vi "Parse String.vi"(8 "error in (no error)":errorcluster, 10 "start at":i32, 11 "TOML String":string) -> (0 "error out":errorcluster, 2 "offset past match":i32, 3 "String":string)   [LabVIEW 2015, in "JSON.lvlib"]
uses:
  JSON.lvlib
  <vilib>/regexp/Match Regular Expression.xnode
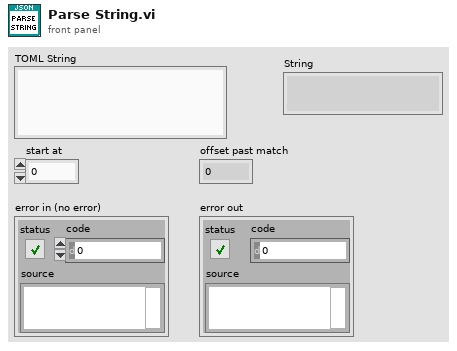
[diagram p1: front panel]
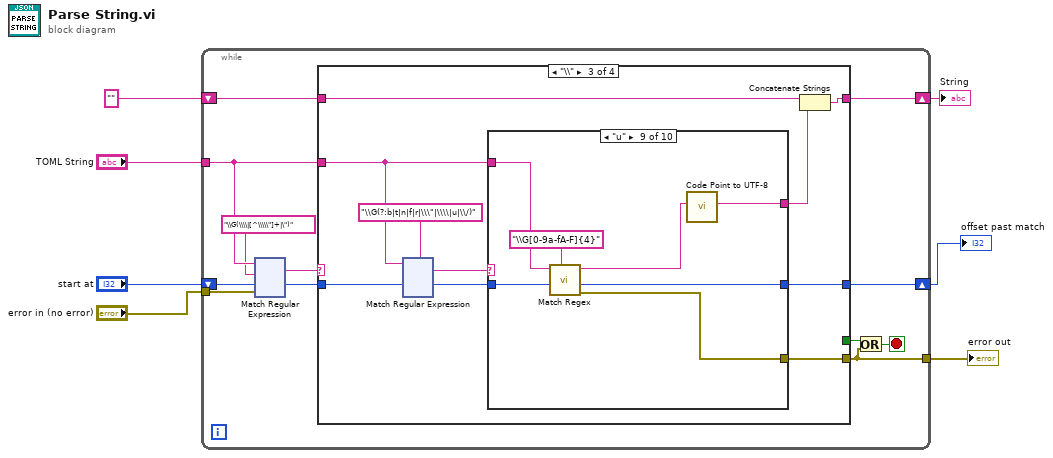
[diagram p0: block diagram]
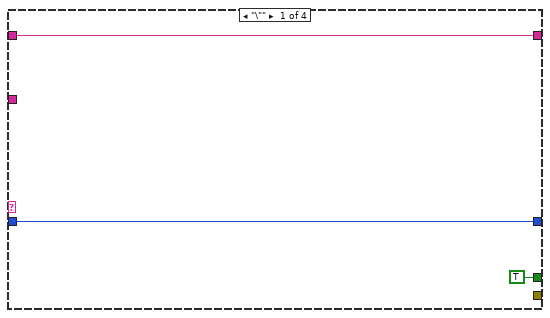
[diagram p2: hidden frame]
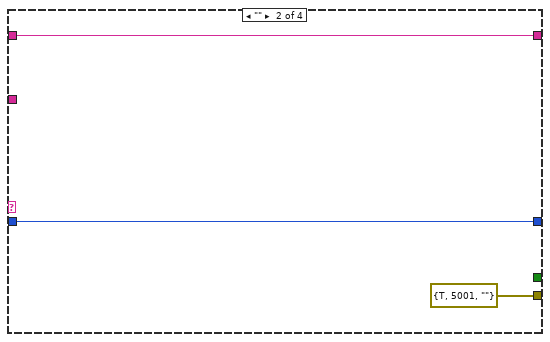
[diagram p3: hidden frame]
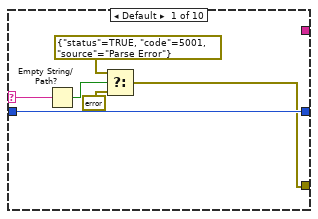
[diagram p4: hidden frame]
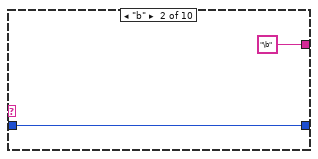
[diagram p5: hidden frame]
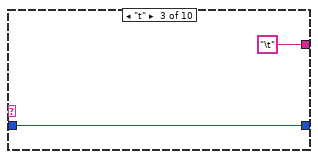
[diagram p6: hidden frame]
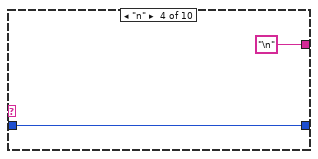
[diagram p7: hidden frame]
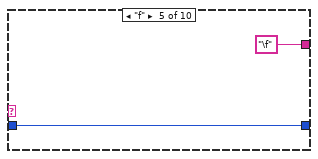
[diagram p8: hidden frame]
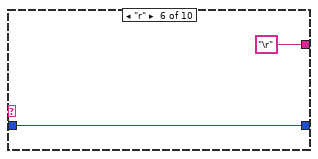
[diagram p9: hidden frame]
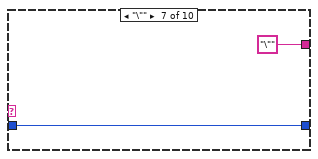
[diagram p10: hidden frame]
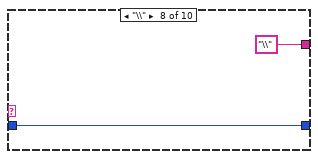
[diagram p11: hidden frame]
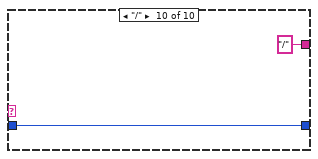
[diagram p12: hidden frame]
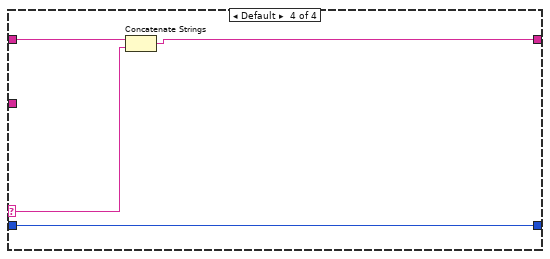
[diagram p13: hidden frame]
diagram:
  n1 = while {
    tunnel: "error in (no error)" -> [w19]
    tunnel: "TOML String" -> [w12]
    shift-right: [w17] -> w3
    shift-left: "start at" -> [w18]
    shift-right: [w15] -> w4
    shift-left: "" -> [w14]
    tunnel: [w10] -> w5
    stop <- w11 stop-if-true
    n2 = xnode "Match Regular Expression"("input string"=w12, "regular expression"="\\G(\\\\|[^\\\\\"]+|\")", "offset (0)"=w18, "error in"=w19) -> ("whole match"=w9:string, "offset past match"=w16:i32)  [unwired: 2 in, 3 out]
    n3 = case shown="\"\\\\\"" w9 {
      selector: w9 -> [_ _ _ w181]
      tunnel: [w21 w24 w31 w182] -> w17
      tunnel: w16 -> [w21 w24 w34 w182]
      tunnel: [w22 w25 w29 w179] -> w15
      tunnel: w14 -> [w22 w25 w35 w180]
      tunnel: [TRUE _ _ _] -> w13
      tunnel: w12 -> [_ _ w27 _]
      tunnel: [_ errorcluster {"status"=TRUE, "code"=5001, "source"=""} ("error constant") w32 _] -> w10
      frame "\"" {
      }
      frame "" {
      }
      frame "\\" {
        n4 = xnode "Match Regular Expression"("input string"=w27, "regular expression"="\\G(?:b|t|n|f|r|\\\"|\\\\|u|\\/)", "offset (0)"=w34) -> ("whole match"=w26:string, "offset past match"=w30:i32)  [unwired: 3 in, 3 out]
        n5 = case shown="\"u\"" w26 {
          selector: w26 -> [w40 _ _ _ _ _ _ _ _ _]
          tunnel: [w36 _ _ _ _ _ _ _ w59 _] -> w32
          tunnel: [w41 w42 w44 w46 w48 w50 w52 w54 w60 w63] -> w31
          tunnel: w30 -> [w41 w42 w44 w46 w48 w50 w52 w54 w61 w63]
          tunnel: [_ "\b" ("regular expression") "\t" ("regular expression") "\n" ("regular expression") "\f" ("regular expression") "\r" ("regular expression") "\"" ("regular expression") "\\" ("regular expression") w57 "/" ("UTF-8")] -> w28
          tunnel: w27 -> [_ _ _ _ _ _ _ _ w62 _]
          frame Default {
            n6 = Empty String/Path?(string/path=w40) -> (empty?=w39:bool)
            n7 = Select(t=errorcluster {"status"=TRUE, "code"=5001, "source"="Parse Error"} ("error constant"), s=w39, f=errorcluster {"status"=FALSE, "code"=0, "source"=""}) -> (s? t:f=w36:errorcluster)
          }
          frame "b" {
          }
          frame "t" {
          }
          frame "n" {
          }
          frame "f" {
          }
          frame "r" {
          }
          frame "\"" {
          }
          frame "\\" {
          }
          frame "u" {
            n8 = call "Match Regex.vi"("regular expression"="\\G[0-9a-fA-F]{4}", "offset"=w61, "String"=w62) -> ("error out"=w59:errorcluster, "offset past match"=w60:i32, "whole match"=w56:string)  [unwired: 5 in, 1 out]
            n9 = call "Code Point to UTF-8.vi"("Code Point"=w56) -> ("UTF-8"=w57:string)  [unwired: 10 in]
          }
          frame "/" {
          }
        }
        n10 = Concatenate Strings(w35, w28) -> (w29:string)
      }
      frame Default {
        n11 = Concatenate Strings(w180, w181) -> (w179:string)
      }
    }
    n12 = Or(x=w13, y=w10) -> (x .or. y?=w11:bool)
  }
  "error out" <- w5
  "offset past match" <- w3
  "String" <- w4
